vi "Write Lane Length (mm).vi"(8 "error in (no error)":errorcluster, 10 "Lane Length (mm)":dbl, 11 "Stage Controller in":refnum<class "Stage Controller.lvclass">) -> (0 "error out":errorcluster, 3 "Stage Controller out":refnum<class "Stage Controller.lvclass">)   [LabVIEW 2015, in "Stage Controller.lvlib" / "Stage Controller.lvclass"]
uses:
  Stage Controller.lvclass
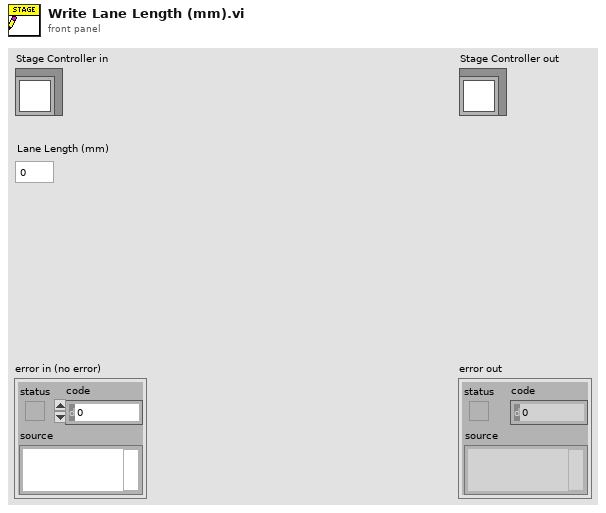
[diagram p1: front panel]
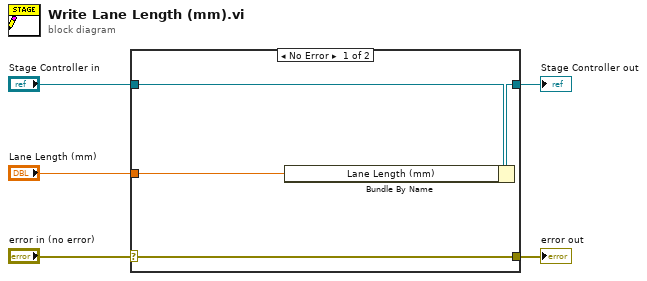
[diagram p0: block diagram]
diagram:
  n1 = case shown="No Error" "error in (no error)" {
    selector: "error in (no error)" -> [w9 w10]
    tunnel: [w9 w10] -> w4
    tunnel: [w7 w11] -> w2
    tunnel: "Stage Controller in" -> [w8 w11]
    tunnel: "Lane Length (mm)" -> [w6 _]
    frame No Error {
      n2 = Bundle By Name(cluster=w8, "Lane Length (mm)"=w6) -> (w7:refnum<class "Stage Controller.lvclass">)
    }
    frame Error {
    }
  }
  "error out" <- w4
  "Stage Controller out" <- w2
